vi "Data.Config, Load Test Limits from XML File.vi"(8 "error in (no error)":errorcluster, 11 "Limit File Path":path) -> (0 "error out":errorcluster, 1 "Limits":T1[](array[typedef])=[{"Name"="asv", "LimType"=enum."None", "LL"=1234.0, "UL"=1234.0, "Units"="", "FailCode"=0, "FailDesc"=""}, {"Name"=", kjh/lk", "LimType"=enum."None", "LL"=1234.0, "UL"=1234.0, "Units"="", "FailCode"=0, "FailDesc"=""}], 2 "File Version":string, 3 "File Name":string, 4 "Limits in Variant":variant)   [LabVIEW 2024, in "EQMF.lvlib" / "Data.lvlib"]
uses:
  Data.lvlib
  Files/File Utils.lvlib
  TypeDefs/Data.Result Limit XML File Data.ctl
  TypeDefs/Data.Result Numeric Limit Type.ctl
  TypeDefs/Data.Result Limit Definition.ctl
  Status/Status Utils.lvlib
panel:
  out "Test Name":string
  out "XML Version":string
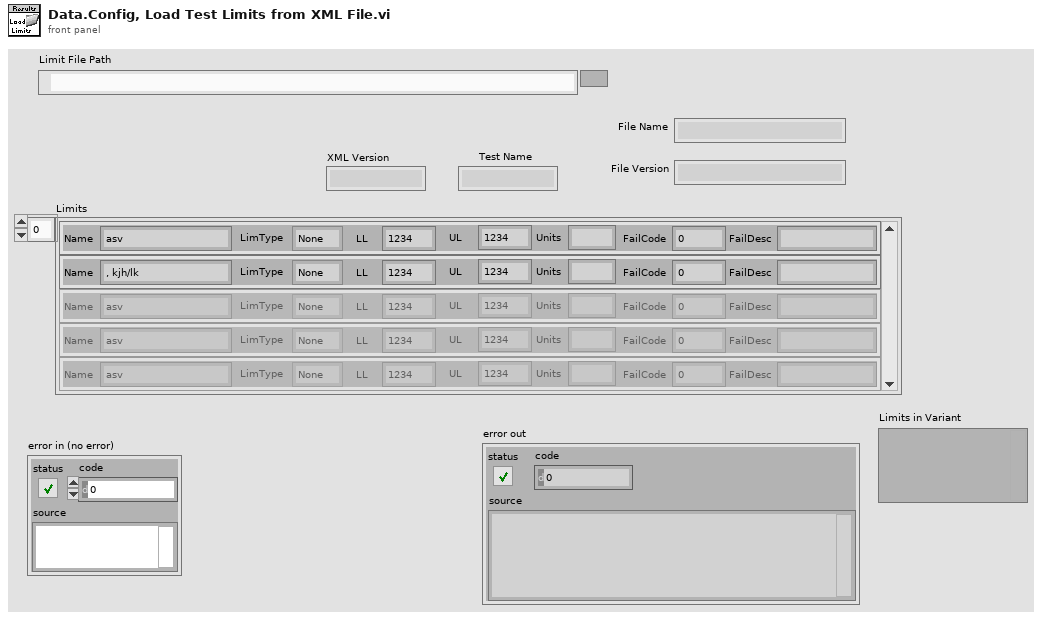
[diagram p1: front panel]
types:
  T1 = typedef "EQMF.lvlib/Data.lvlib/Data.Result Limit Definition.ctl" = cluster{"Name":string, "LimType":T2, "LL":dbl, "UL":dbl, "Units":string, "FailCode":i32, "FailDesc":string}
  T2 = typedef "EQMF.lvlib/Data.lvlib/Data.Result Numeric Limit Type.ctl" = enum16{"None", "EQ", "NE", "GT", "LT", "GE", "LE", "GTLT", "GELE", "GELT", "GTLE", "LTGT", "LEGE", "LEGT", "LTGE"}
  T3 = typedef "EQMF.lvlib/Data.lvlib/Data.Result Limit XML File Data.ctl" = cluster{"#attributes":cluster{"XMLFormatVer":string}, "TestName":string, "FileVersion":string, "Limit":T1[]}
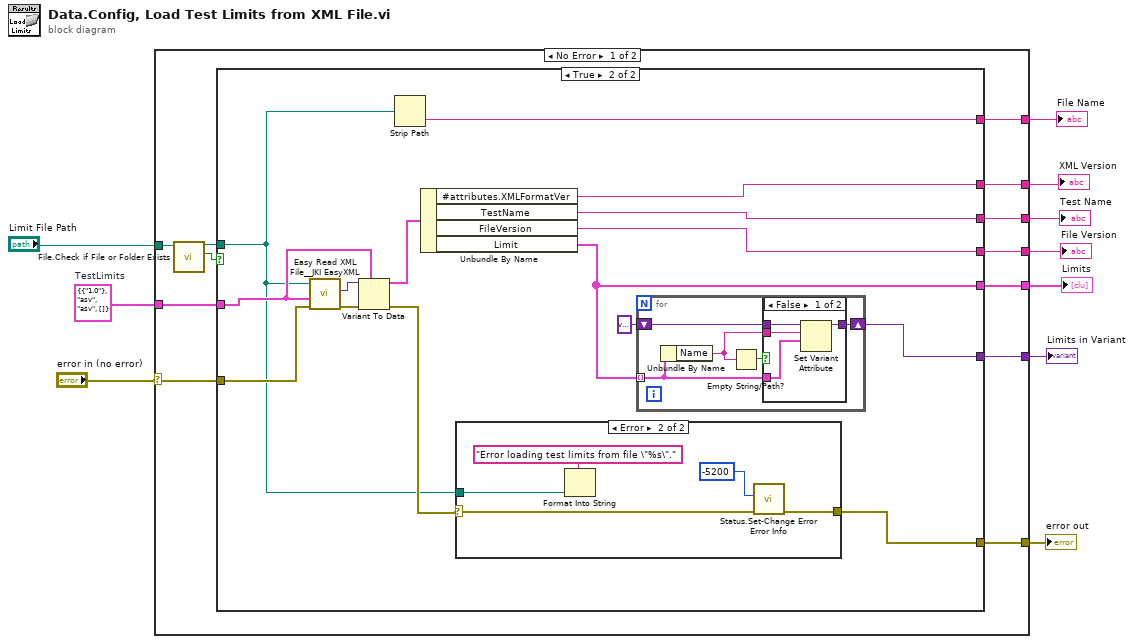
[diagram p0: block diagram]
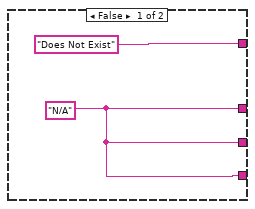
[diagram p2: hidden frame]
diagram:
  w10 = T3 {"#attributes"={"XMLFormatVer"="1.0"}, "TestName"="asv", "FileVersion"="asv", "Limit"=[]}  # TestLimits
  n1 = case shown="No Error" "error in (no error)" {
    selector: "error in (no error)" -> [w15 w56]
    tunnel: w10 -> [w22 _]
    tunnel: [w21 _] -> w9
    tunnel: [w20 _] -> w8
    tunnel: [w19 _] -> w7
    tunnel: [w18 _] -> w6
    tunnel: [w17 _] -> w5
    tunnel: [w16 _] -> w4
    tunnel: [w14 w56] -> w2
    tunnel: "Limit File Path" -> [w12 _]
    frame No Error {
      n2 = call "File.Check if File or Folder Exists.vi"("Path"=w12) -> ("Exists"=w11:bool, "Dup Path"=w13:path)  [unwired: 6 in, 3 out]
      n3 = case shown="True" w11 {
        tunnel: w22 -> [_ w36]
        tunnel: [w23 w35] -> w21
        tunnel: [w23 w34] -> w20
        tunnel: [w23 w33] -> w19
        tunnel: ["Does Not Exist" w32] -> w18
        tunnel: [_ w31] -> w17
        tunnel: [_ w29] -> w16
        tunnel: w15 -> [_ w28]
        tunnel: [_ w26] -> w14
        tunnel: w13 -> [_ w25]
        frame False {
          w23 = "N/A"
        }
        frame True {
          n4 = call <vilib>:"Easy Read XML File__JKI EasyXML.vi"("error in (no error)"=w28, "LabVIEW Data (Type)"=w36, "XML File Path"=w25) -> ("error out"=w39:errorcluster, "LabVIEW Data"=w38:variant)  [unwired: 6 in, 1 out]
          n5 = Variant To Data(error in=w39, type=w36, Variant=w38) -> (data=w37:T3, error out=w27:errorcluster)
          n6 = Strip Path(path=w25) -> (name=w32:string)  [unwired: 1 out]
          n7 = Unbundle By Name(w37) -> ("#attributes.XMLFormatVer"=w35:string, "TestName"=w34:string, "FileVersion"=w33:string, "Limit"=w31:T1[])
          n8 = case shown="Error" w27 {
            selector: w27 -> [w40 w45]
            tunnel: [w40 w43] -> w26
            tunnel: w25 -> [_ w41]
            frame No Error {
            }
            frame Error {
              n9 = Format Into String(format string="Error loading test limits from file \"%s\".", w41) -> ()  [unwired: 2 in, 2 out]
              n10 = call "Status.Set-Change Error Error Info.vi"("Error In"=w45, "NewCode"=-5200 ("code")) -> ("Error Out"=w43:errorcluster)  [unwired: 9 in]
            }
          }
          n11 = for {
            tunnel: w31 -> [w48] mode=indexing
            shift-right: [w49] -> w29
            shift-left: variant ("Limits in Variant") -> [w50]
            n12 = Unbundle By Name(w48) -> ("Name"=w47:string)
            n13 = Empty String/Path?(string/path=w47) -> (empty?=w46:bool)
            n14 = case shown="False" w46 {
              tunnel: w50 -> [w54 w55]
              tunnel: [w53 w55] -> w49
              tunnel: w48 -> [w52 _]
              tunnel: w47 -> [w51 _]
              frame False {
                n15 = Set Variant Attribute(Variant=w54, name=w51, value=w52) -> (Variant out=w53:variant)  [unwired: 1 in, 2 out]
              }
              frame True {
              }
            }
          }
        }
      }
    }
    frame Error {
    }
  }
  "Limits" <- w5
  "XML Version" <- w9
  "File Name" <- w6
  "File Version" <- w7
  "Test Name" <- w8
  "Limits in Variant" <- w4
  "error out" <- w2
